vi "run_model.vi"(8 "error in (no error)":errorcluster, 11 "Image Paths":string[](array[string])) -> (0 "error out":errorcluster, 3 "Results path":path=path "C:/Users/G Malone/Documents/RailTechnology/VIs/images.csv")   [LabVIEW 2023]
uses:
  <vilib>/Utility/file.llb/Write Delimited Spreadsheet (string).vi
panel:
  out "return code":i32
  out "time (ms)":u32
  out "standard output":string
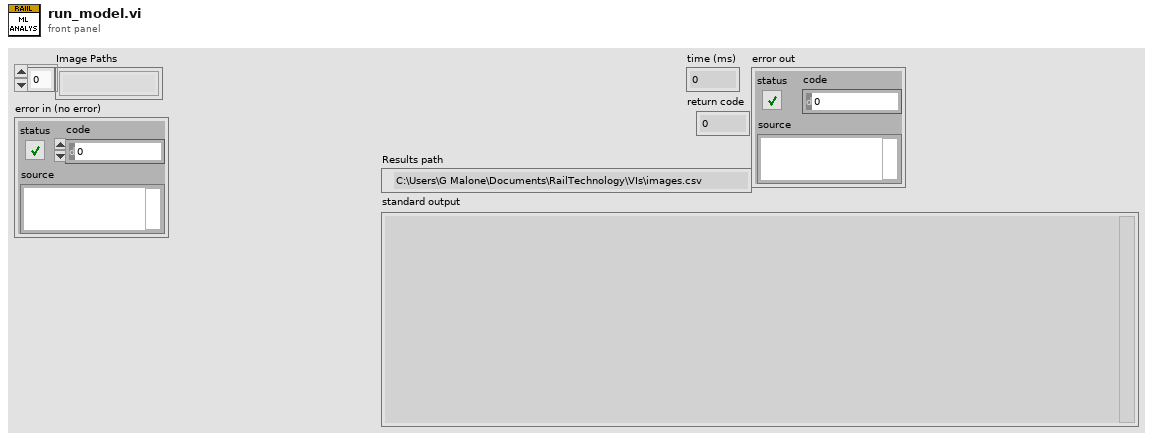
[diagram p1: front panel]
types:
  T1 = enum16{"open", "replace", "create", "open or create", "replace or create", "replace or create with confirmation"}
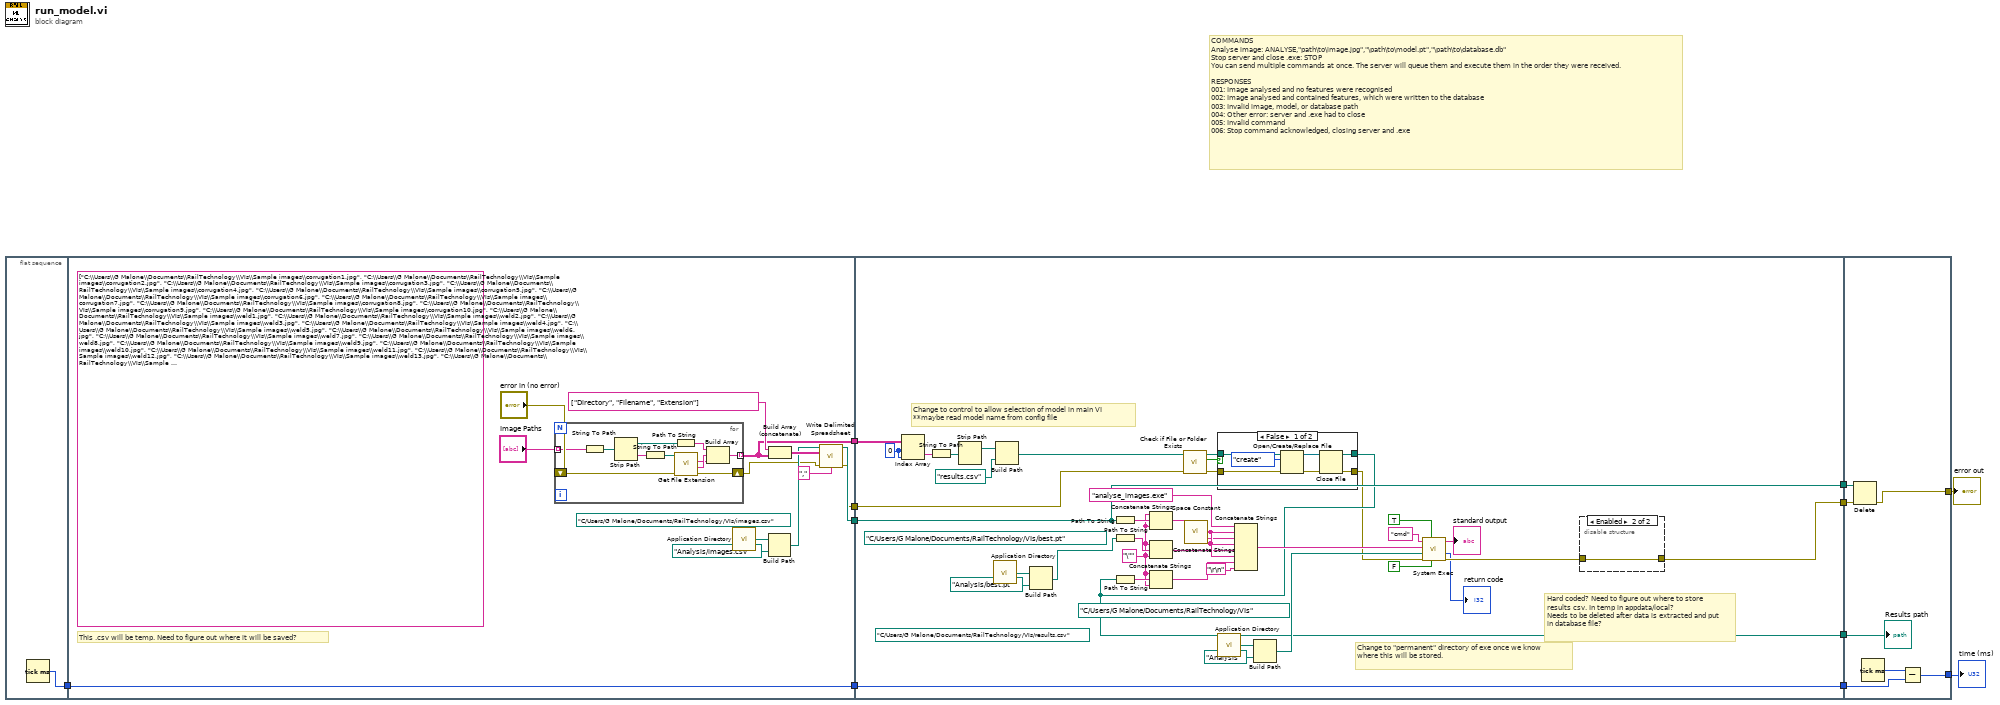
[diagram p0: block diagram]
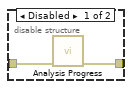
[diagram p2: hidden frame]
diagram:
  # "COMMANDS\nAnalyse image: ANALYSE,\"path\\to\\image.jpg\",\"\\path\\to\\model.pt\",\"\\path\\to\\database.db\"\nStop server and close .exe: STOP\nYou can send multiple commands at once. The server will queue them and execute them in the order they were received.\n\nRESPONSES\n001: Image analysed and no features were recognised\n002: Image analysed and contained features, which were written to the database\n003: Invalid image, model, or database path\n004: Other error: server and .exe had to close\n005: Invalid command\n006: Stop command acknowledged, closing server and .exe"
  n1 = flat-sequence {
    tunnel: [w12] -> w3
    tunnel: [w18] -> w11
    tunnel: [w17] -> w8
    tunnel: [w15] -> w7
    tunnel: w3 -> [w13]
    tunnel: [w13] -> w2
    tunnel: w11 -> [w64]
    tunnel: [w40] -> w10
    tunnel: [w64] -> w9
    tunnel: w8 -> [w54]
    tunnel: w7 -> [w38]
    tunnel: [w37] -> w6
    tunnel: w2 -> [w51]
    tunnel: [w51] -> w1
    tunnel: w10 -> [w94]
    tunnel: w9 -> [w93]
    tunnel: w6 -> [w92]
    tunnel: [w91] -> w5
    tunnel: [w89] -> w4
    tunnel: w1 -> [w88]
    frame #0 {
      n2 = Tick Count (ms)() -> (millisecond timer value=w12:u32)
    }
    frame #1 {
      (unwired) path "C:/Users/G Malone/Documents/RailTechnology/VIs/images.csv" ("file path (dialog if empty)")
      (unwired) string[] ["C:\\Users\\G Malone\\Documents\\RailTechnology\\VIs\\Sample images\\corrugation1.jpg", "C:\\Users\\G Malone\\Documents\\RailTechnology\\VIs\\Sample images\\corrugation2.jpg", "C:\\Users\\G Malone\\Documents\\RailTechnology\\VIs\\Sample images\\corrugation3.jpg", "C:\\Users\\G Malone\\Documents\\RailTechnology\\VIs\\Sample images\\corrugation4.jpg", "C:\\Users\\G Malone\\Documents\\RailTechnology\\VIs\\Sample images\\corrugation5.jpg", "C:\\Users\\G Malone\\Documents\\RailTechnology\\VIs\\Sample images\\corrugation6.jpg", "C:\\Users\\G Malone\\Documents\\RailTechnology\\VIs\\Sample images\\corrugation7.jpg", "C:\\Users\\G Malone\\Documents\\RailTechnology\\VIs\\Sample images\\corrugation8.jpg", "C:\\Users\\G Malone\\Documents\\RailTechnology\\VIs\\Sample images\\corrugation9.jpg", "C:\\Users\\G Malone\\Documents\\RailTechnology\\VIs\\Sample images\\corrugation10.jpg", "C:\\Users\\G Malone\\Documents\\RailTechnology\\VIs\\Sample images\\weld1.jpg", "C:\\Users\\G Malone\\Documents\\RailTechnology\\VIs\\Sample images\\weld2.jpg", "C:\\Users\\G Malone\\Documents\\RailTechnology\\VIs\\Sample images\\weld3.jpg", "C:\\Users\\G Malone\\Documents\\RailTechnology\\VIs\\Sample images\\weld4.jpg", "C:\\Users\\G Malone\\Documents\\RailTechnology\\VIs\\Sample images\\weld5.jpg", "C:\\Users\\G Malone\\Documents\\RailTechnology\\VIs\\Sample images\\weld6.jpg", "C:\\Users\\G Malone\\Documents\\RailTechnology\\VIs\\Sample images\\weld7.jpg", "C:\\Users\\G Malone\\Documents\\RailTechnology\\VIs\\Sample images\\weld8.jpg", "C:\\Users\\G Malone\\Documents\\RailTechnology\\VIs\\Sample images\\weld9.jpg", "C:\\Users\\G Malone\\Documents\\RailTechnology\\VIs\\Sample images\\weld10.jpg", "C:\\Users\\G Malone\\Documents\\RailTechnology\\VIs\\Sample images\\weld11.jpg", "C:\\Users\\G Malone\\Documents\\RailTechnology\\VIs\\Sample images\\weld12.jpg", "C:\\Users\\G Malone\\Documents\\RailTechnology\\VIs\\Sample images\\weld13.jpg", "C:\\Users\\G Malone\\Documents\\RailTechnology\\VIs\\Sample images\\weld14.jpg", "C:\\Users\\G Malone\\Documents\\RailTechnology\\VIs\\Sample images\\weld15.jpg"]
      # "This .csv will be temp. Need to figure out where it will be saved?"
      n3 = for {
        tunnel: "Image Paths" -> [w36] mode=indexing
        tunnel: [w28] -> w17 mode=indexing
        shift-right: [w26] -> w16
        shift-left: "error in (no error)" -> [w27]
        n4 = String To Path(string=w36) -> (path=w35:path)
        n5 = Strip Path(path=w35) -> (stripped path=w32:path, name=w34:string)
        n6 = String To Path(string=w34) -> (path=w33:path)
        n7 = Path To String(path=w32) -> (string=w31:string)
        n8 = call <vilib>:"Get File Extension.vi"("error in (no error)"=w27, "file"=w33) -> ("error out"=w26:errorcluster, "filename without extension"=w30:string, "lowercase file extension"=w29:string)  [unwired: 5 in, 2 out]
        n9 = Build Array(w31, w30, w29) -> (w28:string[])
      }
      n10 = call <vilib>:"Application Directory.vi"() -> ("Application Directory"=w21:path)
      n11 = Build Path(base path=w21, name or relative path=path "Analysis/images.csv") -> (appended path=w19:path)
      n12 = Build Array (concatenate)(string[] ["Directory", "Filename", "Extension"], w17) -> (w25:string[][])
      n13 = call-poly <vilib>:"Write Delimited Spreadsheet.vi"("file path (dialog if empty)"=w19, "2D data"=w25, "error in (no error)"=w16, "delimiter (\\t)"="," ("delimiter (\\t)")) -> ("new file path (Not A Path if cancelled)"=w18:path, "error out"=w15:errorcluster)  [unwired: 10 in]
    }
    frame #2 {
      w53 = 0 ("index (row)")
      (unwired) path "C:/Users/G Malone/Documents/RailTechnology/VIs/results.csv" ("file path (dialog if empty)")
      (unwired) path "C:/Users/G Malone/Documents/RailTechnology/VIs/best.pt" ("working directory")
      w68 = "\""
      (unwired) path "C:/Users/G Malone/Documents/RailTechnology/VIs" ("working directory")
      # "Hard coded? Need to figure out where to store results csv. In temp in appdata/local?\nNeeds to be deleted after data is extracted and put in database file?"
      # "Change to \"permanent\" directory of exe once we know where this will be stored."
      # "Change to control to allow selection of model in main VI\n**maybe read model name from config file"
      n14 = Index Array(array=w54, index (row)=w53, index (col)=w53) -> (element=w56:string)
      n15 = String To Path(string=w56) -> (path=w55:path)
      n16 = Strip Path(path=w55) -> (stripped path=w52:path)  [unwired: 1 out]
      n17 = call <vilib>:"Application Directory.vi"() -> ("Application Directory"=w62:path)
      n18 = Build Path(base path=w52, name or relative path=path "results.csv") -> (appended path=w41:path)
      n19 = Build Path(base path=w62, name or relative path=path "Analysis/best.pt") -> (appended path=w61:path)
      n20 = Path To String(path=w64) -> (string=w73:string)
      n21 = Path To String(path=w61) -> (string=w71:string)
      n22 = Concatenate Strings(w68, w73, w68) -> (w72:string)
      n23 = Concatenate Strings(w68, w71, w68) -> (w70:string)
      n24 = call <vilib>:"Check if File or Folder Exists.vi"("error in (no error)"=w38, "path"=w41) -> ("error out"=w42:errorcluster, "file or folder exists?"=w44:bool, "dup path"=w43:path)  [unwired: 7 in]
      n25 = call <vilib>:"Space Constant.vi"() -> ("String"=w74:string)
      n26 = case shown="False" w44 {
        tunnel: w43 -> [w85 w87]
        tunnel: w42 -> [w84 w86]
        tunnel: [w80 w87] -> w40
        tunnel: [w79 w86] -> w39
        frame False {
          n27 = Open/Create/Replace File(file path (use dialog)=w85, error in=w84, operation (0:open)=T1."create") -> (refnum out=w81:refnum<file>, error out=w82:errorcluster)  [unwired: 3 in, 1 out]
          n28 = Close File(refnum=w81, error in=w82) -> (path=w80:path, error out=w79:errorcluster)
        }
        frame True {
        }
      }
      n29 = Path To String(path=w40) -> (string=w69:string)
      n30 = Concatenate Strings(w68, w69, w68) -> (w67:string)
      n31 = call <vilib>:"Application Directory.vi"() -> ("Application Directory"=w60:path)
      n32 = Concatenate Strings("analyse_images.exe", w74, w72, w74, w70, w74, w67, "\r\n") -> (w66:string)
      n33 = Build Path(base path=w60, name or relative path=path "Analysis") -> (appended path=w58:path)
      n34 = call <vilib>:"System Exec.vi"("run minimized? (F)"=FALSE, "wait until completion? (T)"=TRUE, "error in (no error)"=w39, "working directory"=w58, "standard input"=w66, "command line"="cmd") -> ("error out"=w46:errorcluster, "return code"=→"return code":i32, "standard output"=→"standard output":string)  [unwired: 2 in, 1 out]
      n35 = disable-structure shown="Enabled" {
        disable-tunnel: w46 -> [w77 w78]
        disable-tunnel: [w76 w78] -> w37
        frame Disabled {
          n36 = call "Analysis Progress.vi"("error in (no error)"=w77) -> ("error out"=w76:errorcluster)  [unwired: 10 in]
        }
        frame Enabled {
        }
      }
    }
    frame #3 {
      n37 = Delete(path (use dialog)=w93, error in=w92) -> (error out=w91:errorcluster)  [unwired: 3 in, 2 out]
      n38 = Tick Count (ms)() -> (millisecond timer value=w90:u32)
      n39 = Subtract(x=w90, y=w88) -> (x-y=w89:u32)
      "Results path" <- w94
    }
  }
  "error out" <- w5
  "time (ms)" <- w4
